vi "Main_Playground.vi"() -> ()   [LabVIEW 2017]
panel:
  in  "Take Data":bool
  in  "Calibrate":bool
  in  "stop":bool
  in  "OK Button":bool
  in  "Manually Load VI":path
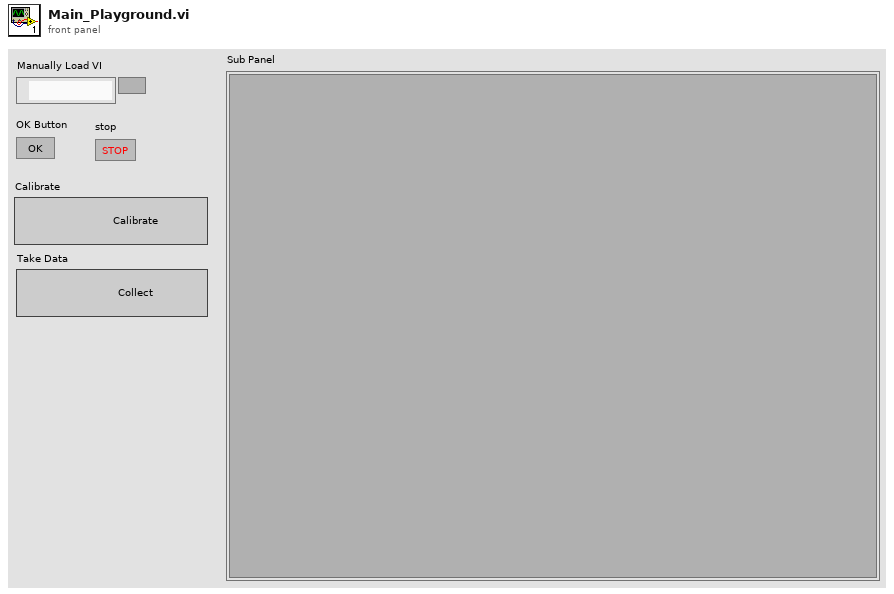
[diagram p1: front panel]
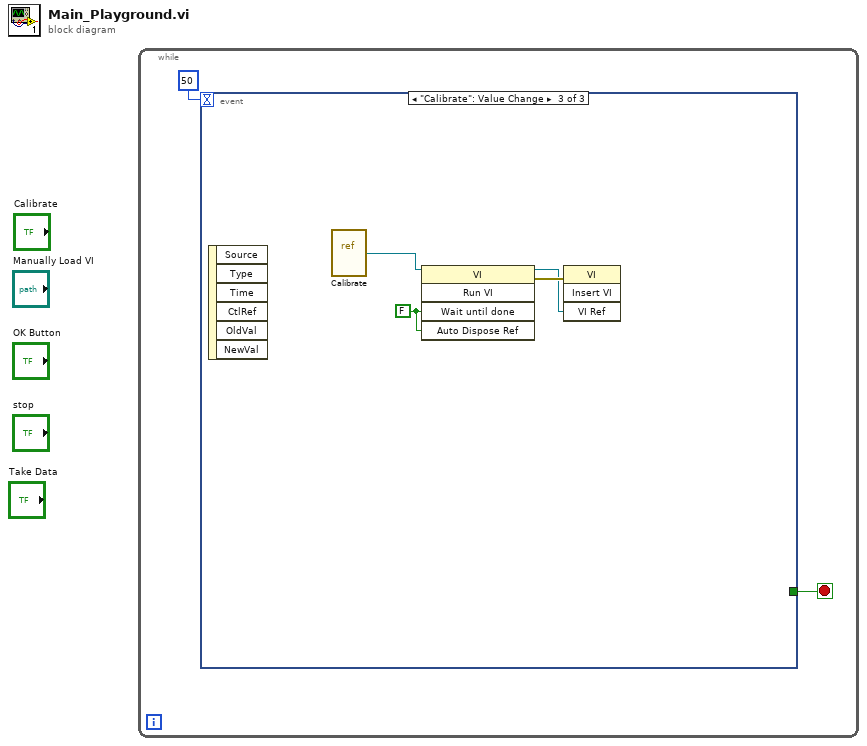
[diagram p0: block diagram]
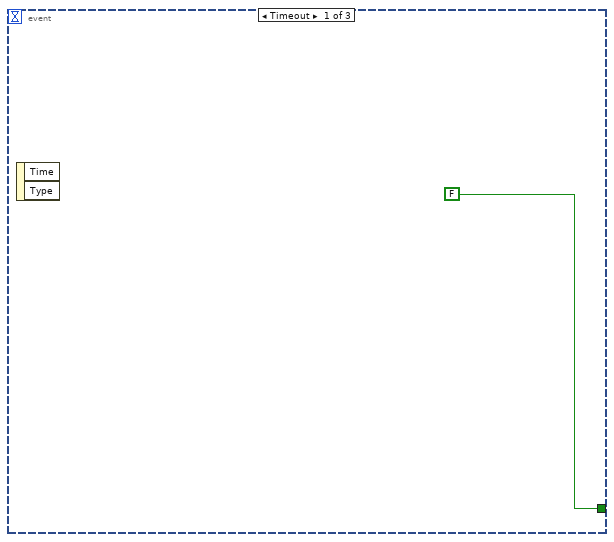
[diagram p2: hidden frame]
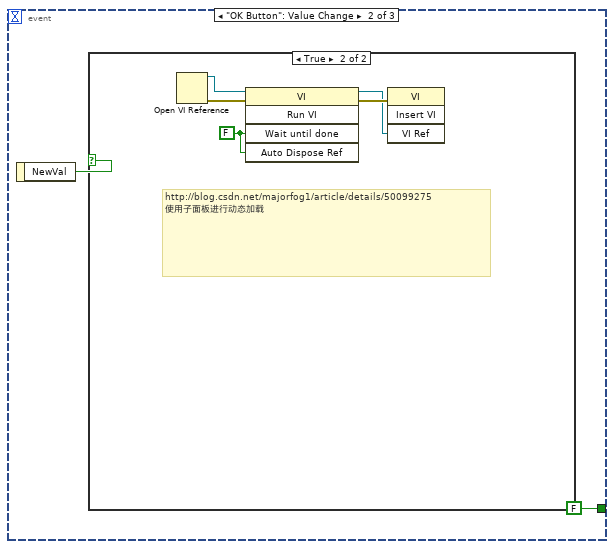
[diagram p3: hidden frame]
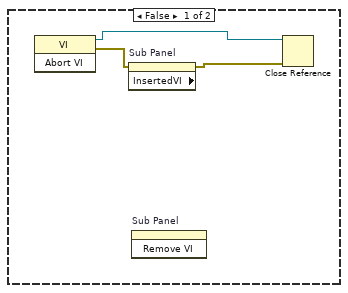
[diagram p4: hidden frame]
diagram:
  n1 = while {
    stop <- w1 stop-if-true
    n2 = event shown="[2] \"Calibrate\": Value Change" {
      selector: _ -> [_ _ _]
      dyn-events: _ -> [_ _ _]
      timeout: 50 -> [_ _ _]
      tunnel: [FALSE FALSE _] -> w1
      event Timeout {
        n3 = event-data() -> ()  [unwired: 1 in, 2 out]
      }
      event "OK Button": Value Change {
        n4 = event-data() -> ("NewVal"=w5:bool)  [unwired: 1 in]
        n5 = case shown="True" w5 {
          frame False {
            n6 = invoke class="VI" method="Abort VI"() -> (reference out=w8:refnum<vi>, error out=w7:errorcluster)  [unwired: 3 in, 1 out]
            n7 = property on="Sub Panel" class="SubPnl" props=["InsertedVI"](error in=w7) -> (error out=w6:errorcluster)  [unwired: 1 in, 2 out]
            n8 = invoke on="Sub Panel" class="SubPnl" method="Remove VI"() -> ()  [unwired: 3 in, 3 out]
            n9 = Close Reference(reference=w8, error in (no error)=w6) -> ()  [unwired: 1 out]
          }
          frame True {
            w11 = FALSE
            # "http://blog.csdn.net/majorfog1/article/details/50099275\n使用子面板进行动态加载"
            n10 = Open VI Reference() -> (vi reference=w10:refnum<vi>, error out=w12:errorcluster)  [unwired: 6 in]
            n11 = invoke class="VI" method="Run VI"(reference=w10, error in=w12, "Wait until done"=w11, "Auto Dispose Ref"=w11) -> (reference out=w9:refnum<vi>, error out=w13:errorcluster)  [unwired: 1 in, 3 out]
            n12 = invoke on="Invoke Node" class="VI" method="Insert VI"(error in=w13, "VI Ref"=w9) -> ()  [unwired: 2 in, 4 out]
          }
        }
      }
      event "Calibrate": Value Change {
        w16 = FALSE
        n13 = event-data() -> ()  [unwired: 1 in, 6 out]
        n14 = vi-ref "Calibrate.vi"() -> (w14:refnum<vi>)
        n15 = invoke class="VI" method="Run VI"(reference=w14, "Wait until done"=w16, "Auto Dispose Ref"=w16) -> (reference out=w15:refnum<vi>, error out=w17:errorcluster)  [unwired: 2 in, 3 out]
        n16 = invoke on="Invoke Node" class="VI" method="Insert VI"(error in=w17, "VI Ref"=w15) -> ()  [unwired: 2 in, 4 out]
      }
    }
  }
